vi "BundleCommData.vi"(8 "error in (no error)":errorcluster, 10 "received_data":string, 11 "send_data":string) -> (0 "error out":errorcluster, 3 "communication_data":T1)   [LabVIEW 2020, in "OXYGEN_Datastream.lvlib"]
uses:
  OXYGEN_Datastream.lvlib
  TypeDefs/Cluster_RawCommData.ctl
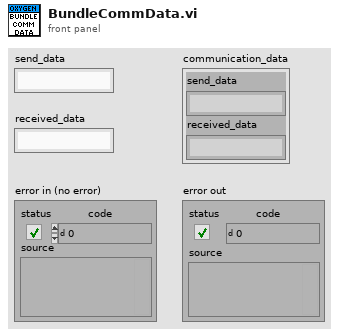
[diagram p1: front panel]
types:
  T1 = typedef "OXYGEN_Datastream.lvlib/Cluster_RawCommData.ctl" = cluster{"send_data":string, "received_data":string}
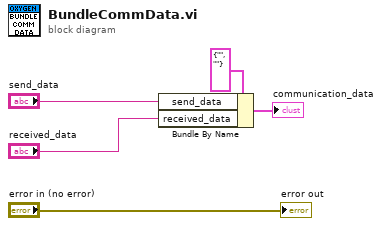
[diagram p0: block diagram]
diagram:
  n1 = Bundle By Name(cluster=T1 {"send_data"="", "received_data"=""} ("communication_data"), "send_data"="send_data", "received_data"="received_data") -> (→"communication_data":T1)
  "error out" <- "error in (no error)"
